vi "ziExample-Module-Impedance.vi"() -> ()   [LabVIEW 2009]
doc: "Control a Zurich instrument device via the LabOne Labview API. \nRequirements: Zurich Instruments MFLI+IA/ MFIA\nThis example shows how to use retrieve impedance data and utilize the sweeper.\n\n© Zurich Instruments AG, www.zhinst.com"
uses:
  <instrlib>/Zurich Instruments LabOne/Public/Modules/ziTypeModSweeperImpedanceWave.ctl
  <instrlib>/Zurich Instruments LabOne/Public/Modules/ziModSetValueDouble.vi
  <instrlib>/Zurich Instruments LabOne/Public/Modules/ziModSetValueBinary.vi
  <instrlib>/Zurich Instruments LabOne/Public/Modules/ziModSetValueDoubleArray.vi
  <instrlib>/Zurich Instruments LabOne/Public/Configure/ziSetValueDoubleArray.vi
  <instrlib>/Zurich Instruments LabOne/Public/Modules/ziModGetSweeperData.vi
  <instrlib>/Zurich Instruments LabOne/Public/Data/ziGetEventImpSample.vi
  <instrlib>/Zurich Instruments LabOne/Zurich Instruments LabOne.lvlib
panel:
  out "ImpedanceSweeperData":T1 {"bandwidthMode" format="%f"; "flags" format="%f"; "sampleFormat" format="%f"; "sweepMode" format="%f"; "sampleCount" format="%f"; "timestamp" format="%f"}
  out "param1":dbl[](array[numeric])
  out "param0":dbl[](array[numeric])
  in  "stop":bool
  out "Param1":dbl
  out "Param0":dbl format="%#_6p"
  out "Error Out":errorcluster
  in  "Address":string="DEV"
  out "Selected Device":string
  in  "subscribepath":string="imps/0/sample" caption="Subscribe Path"
  in  "moduleID":u16(ring) items=["sweep", "zoomFFT", "deviceSettings", "record", "pllAdvisor", "pidAdvisor"]
  out "Param1":cluster{"grid":dbl[], "r_avg":dbl[]}(graph)
  out "Param 0":cluster{"grid":dbl[], "r_avg":dbl[]}(graph)
  # "ziExample-IMPModul.vi\nRequirements: MFLI + IA / MFIA\nsee block diagram for VI description"
  # "Tested Devices:\n\n- MFLI"
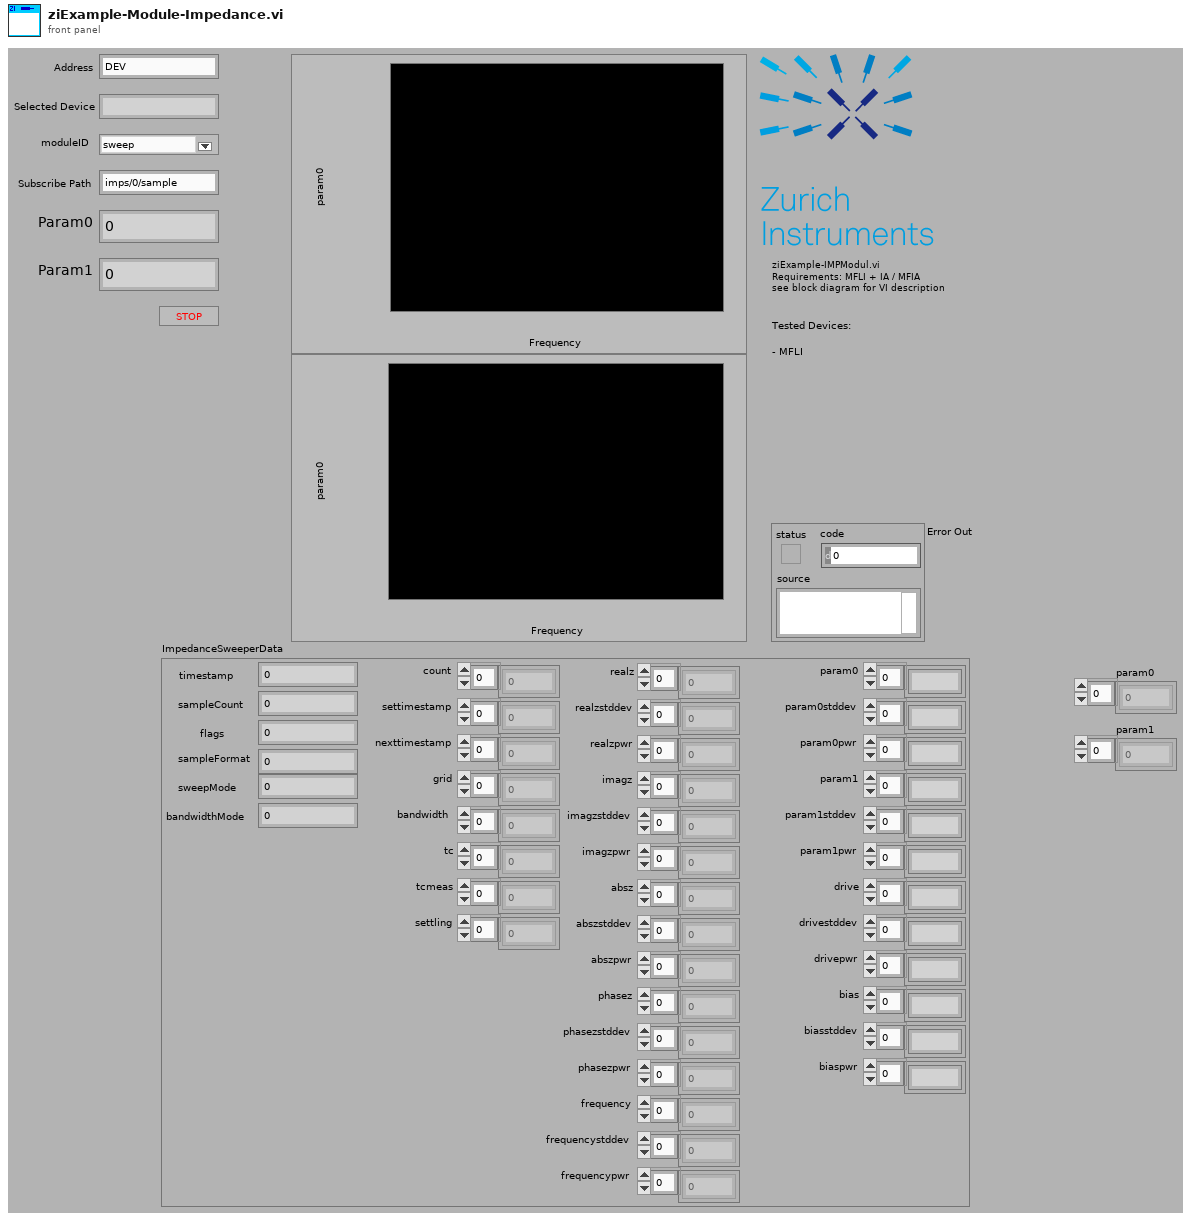
[diagram p1: front panel]
types:
  T1 = typedef "Zurich Instruments LabOne.lvlib/ziTypeModSweeperImpedanceWave.ctl" = cluster{"timestamp":u64, "sampleCount":u64, "flags":u8, "sampleFormat":u8, "sweepMode":u8, "bandwidthMode":u8, "count":u64[], "settimestamp":u64[], "nexttimestamp":u64[], "grid":dbl[], "bandwidth":dbl[], "tc":dbl[], "tcmeas":dbl[], "settling":dbl[], "realz":dbl[], "realzstddev":dbl[], "realzpwr":dbl[], "imagz":dbl[], "imagzstddev":dbl[], "imagzpwr":dbl[], "absz":dbl[], "abszstddev":dbl[], "abszpwr":dbl[], "phasez":dbl[], "phasezstddev":dbl[], "phasezpwr":dbl[], "frequency":dbl[], "frequencystddev":dbl[], "frequencypwr":dbl[], "param0":dbl[], "param0stddev":dbl[], "param0pwr":dbl[], "param1":dbl[], "param1stddev":dbl[], "param1pwr":dbl[], "drive":dbl[], "drivestddev":dbl[], "drivepwr":dbl[], "bias":dbl[], "biasstddev":dbl[], "biaspwr":dbl[]}
  T2 = typedef "Zurich Instruments LabOne.lvlib/ziTypeHandle.ctl" = cluster{"handleValid":bool, "Conn":u64, "Path Prefix":string, "Handle":u64, "Connected":bool, "Clockbase(s)":dbl}
  T3 = typedef "Zurich Instruments LabOne.lvlib/ziTypeModHandle.ctl" = cluster{"handleValid":bool, "Conn":u64, "ModHandle":u64, "moduleID":string, "Path Prefix":string}
  T4 = typedef "Zurich Instruments LabOne.lvlib/ziTypeModResults.ctl" = cluster{"PathArray":string[], "ValueType":T5, "NoOfResults":u64, "HeaderType":enum16{"HEADER_TYPE_NONE", "HEADER_TYPE_SWTRIGGER", "HEADER_TYPE_SWEEPER"}, "ziSWTriggerHeader":T6[], "ziSweeperHeader":T7[]}
  T5 = typedef "Zurich Instruments LabOne.lvlib/ziTypePollType.ctl" = enum16{"NONE", "DOUBLE_DATA", "INTEGER_DATA", "DEMOD_SAMPLE", "SCOPE_WAVE_HF2", "AUXIN_SAMPLE", "DIO_SAMPLE", "BYTE_ARRAY", "PWA_WAVE", "9", "10", "11", "12", "13", "14", "15", "TREE_CHANGE_DEPRI", "17", "ERROR", "19", "20", "21", "22", "23", "24", "25", "26", "27", "28", "29", "30", "31", "DOUBLE_DATA_TS", "INTEGER_DATA_TS", "34", "SCOPE_WAVE", "36", "37", "BYTE_ARRAY_TS", "39", "40", "41", "42", "43", "44", "45", "CNT_DATA", "47", "TREE_CHANGE", "49", "50", "51", "52", "53", "54", "55", "56", "57", "58", "59", "60", "61", "62", "63", "SWEEPER_DATA", "SPECTRUM_DATA", "ADVISOR_DATA", "67", "IMP_DATA"}
  T6 = typedef "Zurich Instruments LabOne.lvlib/ziTypeModSWTriggerHeader.ctl" = cluster{"HeaderType":enum8{"HEADER_TYPE_NONE", "HEADER_TYPE_SWTRIGGER", "HEADER_TYPE_SWEEPER"}, "triggerStart":u64, "triggerNumber":u64, "cols":u32, "rows":u32}
  T7 = typedef "Zurich Instruments LabOne.lvlib/ziTypeModSweeperHeader.ctl" = cluster{"HeaderType":enum8{"HEADER_TYPE_NONE", "HEADER_TYPE_SWTRIGGER", "HEADER_TYPE_SWEEPER"}, "sampleFormat":u8}
  T8 = typedef "Zurich Instruments LabOne.lvlib/ziTypeImpedanceSample.ctl" = cluster{"Timestamps (ticks)":u64[], "Z (Ohm)":cdb[], "Freq (Hz)":dbl[], "Osc Phase (deg)":dbl[], "Trigger":u32[], "Param0":dbl[], "Param1":dbl[], "Drive":dbl[], "Bias":dbl[]}
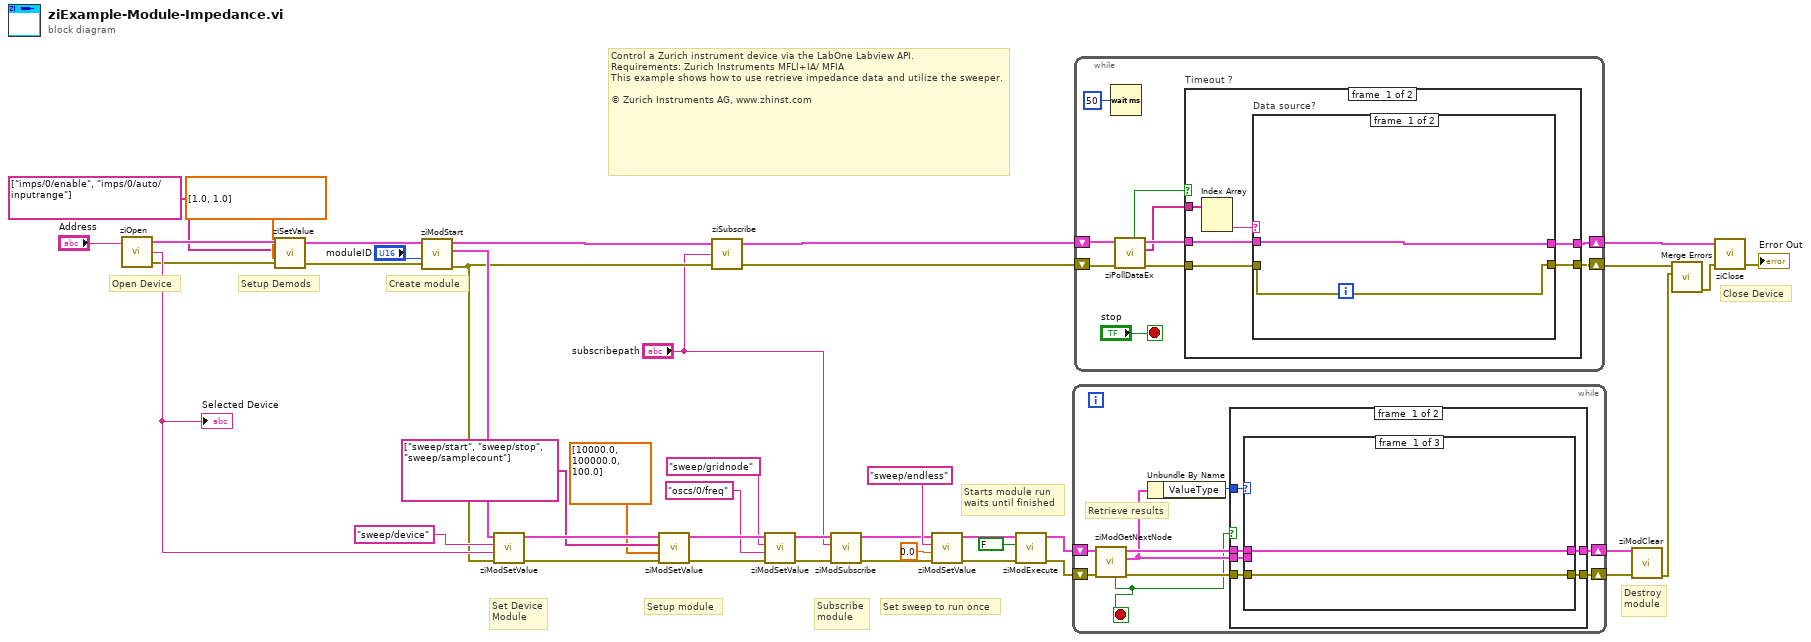
[diagram p0: block diagram]
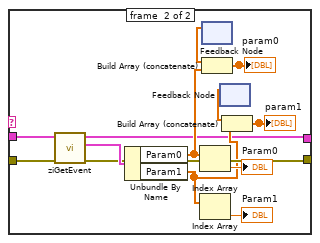
[diagram p2: hidden frame]
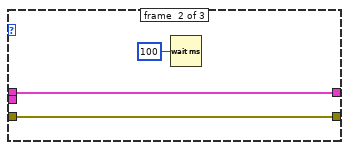
[diagram p4: hidden frame]
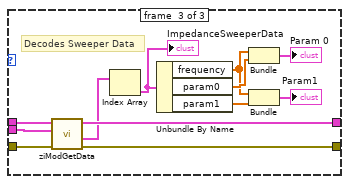
[diagram p5: hidden frame]
diagram:
  # "Control a Zurich instrument device via the LabOne Labview API. \nRequirements: Zurich Instruments MFLI+IA/ MFIA\nThis example shows how to use retrieve impedance data and utilize the sweeper.\n\n© Zurich Instruments AG, www.zhinst.com"
  # "Setup Demods"
  # "Set Device\nModule"
  # "Destroy\nmodule"
  # "Starts module run\nwaits until finished"
  # "Set sweep to run once"
  # "Subscribe\nmodule"
  # "Setup module"
  # "Create module"
  # "Close Device"
  # "Open Device"
  n1 = call <instrlib>:"ziOpen.vi"("Address"="Address") -> ("Error Out"=w21:errorcluster, "Selected Device"=w42:string, "HandleOut"=w24:T2)  [unwired: 1 in, 2 out]
  "Selected Device" <- w42
  n2 = call-poly <instrlib>:"ziSetValue.vi"("Error In"=w21, "Values"=dbl[] [1.0, 1.0], "Paths"=string[] ["imps/0/enable", "imps/0/auto/inputrange"], "Handle In"=w24) -> ("Error Out"=w22:errorcluster, "Handle Out"=w23:T2)  [unwired: 1 in]
  n3 = call <instrlib>:"ziModStart.vi"("Error In"=w22, "module Id"="moduleID", "Handle In"=w23) -> ("Error Out"=w5:errorcluster, "ModHandle Out"=w28:T3, "Handle Out"=w8:T2)  [unwired: 6 in]
  n4 = call-poly <instrlib>:"ziModSetValue.vi"("Error In"=w5, "Data"=w42, "Path"="sweep/device", "ModHandle In"=w28) -> ("Error Out"=w27:errorcluster, "ModHandle Out"=w26:T3)  [unwired: 6 in]
  n5 = call-poly <instrlib>:"ziModSetValue.vi"("Error In"=w27, "Values"=dbl[] [10000.0, 100000.0, 100.0], "Paths"=string[] ["sweep/start", "sweep/stop", "sweep/samplecount"], "ModHandle In"=w26) -> ("Error Out"=w39:errorcluster, "ModHandle Out"=w38:T3)  [unwired: 6 in]
  n6 = call <instrlib>:"ziSubscribe.vi"("error in"=w5, "Path ()"="subscribepath", "Handle In"=w8) -> ("error out"=w6:errorcluster, "Handle Out"=w7:T2)  [unwired: 1 in]
  n7 = call-poly <instrlib>:"ziModSetValue.vi"("Error In"=w39, "Data"="oscs/0/freq", "Path"="sweep/gridnode", "ModHandle In"=w38) -> ("Error Out"=w35:errorcluster, "ModHandle Out"=w41:T3)  [unwired: 6 in]
  n8 = call <instrlib>:"ziModSubscribe.vi"("Error In"=w35, "Path"="subscribepath", "ModHandle In"=w41) -> ("Error Out"=w36:errorcluster, "ModHandle Out"=w37:T3)  [unwired: 6 in]
  n9 = call-poly <instrlib>:"ziModSetValue.vi"("Error In"=w36, "Value"=0.0, "Path"="sweep/endless", "ModHandle In"=w37) -> ("Error Out"=w34:errorcluster, "ModHandle Out"=w33:T3)  [unwired: 6 in]
  n10 = call <instrlib>:"ziModExecute.vi"("Error In"=w34, "Modal (F)"=FALSE ("Modal"), "ziModHandle In"=w33) -> ("Error Out"=w30:errorcluster, "ziModHandle Out"=w32:T3)  [unwired: 5 in, 1 out]
  n11 = while {
    shift-right: [w48] -> w11
    shift-left: w32 -> [w50]
    shift-right: [w47] -> w12
    shift-left: w30 -> [w51]
    stop <- w43 stop-if-true
    # "Retrieve results"
    n12 = call <instrlib>:"ziModGetNextNode.vi"("Error In"=w51, "ModHandle In"=w50) -> ("Error Out"=w44:errorcluster, "ModResults"=w46:T4, "ModHandle Out"=w49:T3, "NoData"=w43:bool)  [unwired: 6 in]
    n13 = Unbundle By Name(w46) -> ("ValueType"=w45:T5)
    n14 = case shown="False" w43 {
      tunnel: w49 -> [w57 w75]
      tunnel: [w56 w75] -> w48
      tunnel: [w55 w76] -> w47
      tunnel: w44 -> [w54 w76]
      tunnel: w46 -> [w53 _]
      tunnel: w45 -> [w52 _]
      frame #0 {
        n15 = case shown="\"SWEEPER_DATA\"" w52 {
          tunnel: w57 -> [w59 w62 w73]
          tunnel: w53 -> [_ _ w74]
          tunnel: w54 -> [w58 w61 w72]
          tunnel: [w58 w61 w71] -> w55
          tunnel: [w59 w62 w70] -> w56
          frame #0 {
          }
          frame #1 {
            n16 = Wait (ms)(milliseconds to wait=u32 100) -> ()  [unwired: 1 out]
          }
          frame #2 {
            # "Decodes Sweeper Data"
            n17 = call-poly <instrlib>:"ziModGetData.vi"("Error In"=w72, "ModResults"=w74, "ModHandle In"=w73) -> ("Error Out"=w71:errorcluster, "SweeperImpedanceWaveArray"=w64:T1[], "ModHandle Out"=w70:T3)  [unwired: 4 in, 2 out]
            n18 = Index Array(array=w64) -> (element=w63:T1)  [unwired: 1 in]
            "ImpedanceSweeperData" <- w63
            n19 = Unbundle By Name(w63) -> ("frequency"=w65:dbl[], "param0"=w69:dbl[], "param1"=w66:dbl[])
            n20 = Bundle("frequency"=w65, "param0"=w69) -> (→"Param 0":cluster{"frequency":dbl[], "param0":dbl[]})  [unwired: 1 in]
            n21 = Bundle("frequency"=w65, "param1"=w66) -> (→"Param1":cluster{"frequency":dbl[], "param1":dbl[]})  [unwired: 1 in]
          }
        }
      }
      frame #1 {
      }
    }
  }
  n22 = while {
    shift-right: [w79] -> w2
    shift-left: w6 -> [w80]
    shift-right: [w83] -> w9
    shift-left: w7 -> [w81]
    stop <- "stop" stop-if-true
    n23 = Wait (ms)(milliseconds to wait=u32 50) -> ()  [unwired: 1 out]
    n24 = call <instrlib>:"ziPollDataEx.vi"("error in"=w80, "Handle In"=w81) -> ("error out"=w82:errorcluster, "PathArray"=w84:string[], "Handle Out"=w85:T2, "Timed Out"=w86:bool)  [unwired: 2 in, 4 out]
    n25 = case "Timeout ?" shown="False" w86 {
      tunnel: w85 -> [w92 w109]
      tunnel: [w91 w109] -> w83
      tunnel: w84 -> [w90 _]
      tunnel: w82 -> [w88 w108]
      tunnel: [w87 w108] -> w79
      frame #0 {
        n26 = Index Array(array=w90) -> (element #2=w89:string)  [unwired: 2 in, 1 out]
        n27 = case "Data source?" shown="\"IMPS\"" w89 {
          tunnel: w92 -> [w94 w107]
          tunnel: [w94 w95] -> w91
          tunnel: w88 -> [w93 w103]
          tunnel: [w93 w102] -> w87
          frame #0 {
          }
          frame #1 {
            n28 = call-poly <instrlib>:"ziGetEvent.vi"("Error In"=w103, "Handle In"=w107) -> ("Error Out"=w102:errorcluster, "Imp Sample Out"=w104:T8, "Handle Out"=w95:T2)  [unwired: 7 in]
            n29 = Unbundle By Name(w104) -> ("Param0"=w101:dbl[], "Param1"=w98:dbl[])
            n30 = Index Array(array=w101) -> (element=→"Param0":dbl)  [unwired: 1 in]
            n31 = Index Array(array=w98) -> (element=→"Param1":dbl)  [unwired: 1 in]
            n32 = feedback #1() -> (w99:dbl[])  [unwired: 1 in]
            n33 = Build Array (concatenate)(w99, w101) -> (w100:dbl[])
            "param0" <- w100
            n34 = feedback #2() -> (w97:dbl[])  [unwired: 1 in]
            n35 = Build Array (concatenate)(w97, w98) -> (w96:dbl[])
            "param1" <- w96
          }
        }
      }
      frame #1 {
        # "Timeout, no action."
      }
    }
  }
  n36 = call <instrlib>:"ziModClear.vi"("Error In"=w12, "ziModHandle In"=w11) -> ("Error Out"=w3:errorcluster)  [unwired: 7 in, 1 out]
  n37 = call <vilib>:"Merge Errors.vi"("error in 2 (no error)"=w3, "error in 1 (no error)"=w2) -> ("error out"=w1:errorcluster)  [unwired: 5 in]
  n38 = call <instrlib>:"ziClose.vi"("Error In"=w1, "Handle In"=w9) -> ("Error Out"=→"Error Out":errorcluster)  [unwired: 2 in, 1 out]
